vi "Memory.Pointer.Parameter Check.Size.0D.vi"(7 "source vi name":string, 8 "error in (no error)":errorcluster, 10 "required size":u64 format="%08x bytes", 11 "Pointer in":refnum<class "Memory.Pointer.lvclass">) -> (0 "error out":errorcluster, 2 "required size out":u64 format="%08x bytes", 3 "Pointer out":refnum<class "Memory.Pointer.lvclass">)   [LabVIEW 2016, in "Memory Manager.lvlib" / "Memory.Pointer.lvclass"]
uses:
  Memory.Pointer.lvclass
  Memory.Pointer.lvclass/Memory.Pointer.ctl
  Memory.Pointer.Errors.Out of Bounds.vi
  Submodules/Static Error Handling/Source/Library/VIs/Static Error Handling.Source Buffer.Write.String.vi
  Memory.Pointer.Errors.Write Pointer Size.vi
  Memory.Pointer.Errors.Create Error.vi
  Submodules/Static Error Handling/Source/Library/VIs/Static Error Handling.Source Buffer.Write.Numeric.Scalar.Base10.vi
  Submodules/Static Error Handling/Source/Library/VIs/Static Error Handling.Source Buffer.Write.Numeric.Scalar.Base10 (U64).vi
  Submodules/Static Error Handling/Source/Library/VIs/Static Error Handling.Error Cluster Constant.vi
  Submodules/Static Error Handling/Source/Library/VIs/Static Error Handling.Error Cluster Constant (256B).vi
  Submodules/Static Error Handling/Source/Library/VIs/Static Error Handling.Parameters.Status.Set.vi
  Submodules/Static Error Handling/Source/Library/VIs/Static Error Handling.Parameters.Code.Set.vi
  Submodules/Static Error Handling/Source/Library/VIs/Static Error Handling.Parameters.VI Source.Set.vi
  Constants/Memory.Constants.vi
  Constants/Memory.Constants.Library Name.vi
  Memory.Pointer.Errors.Get Info.vi
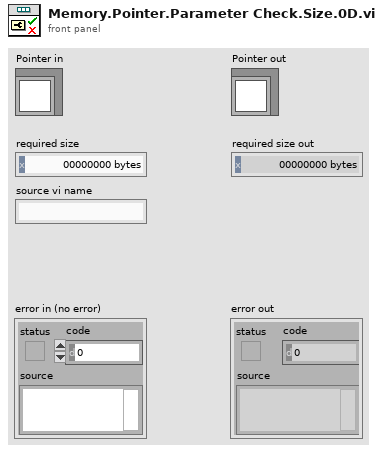
[diagram p1: front panel]
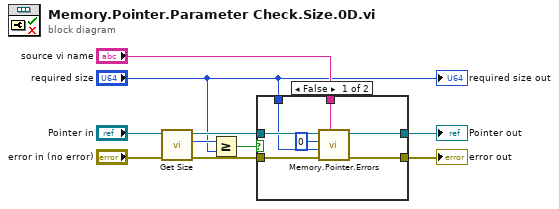
[diagram p0: block diagram]
diagram:
  n1 = call "Get Size.vi"("error in (no error)"="error in (no error)", "Pointer in"="Pointer in") -> ("error out"=w5:errorcluster, "size"=w8:u64, "Pointer out"=w3:refnum<class "Memory.Pointer.lvclass">)  [unwired: 7 in]
  n2 = Greater Or Equal?(x=w8, y="required size") -> (x >= y?=w4:bool)
  n3 = case shown="False" w4 {
    tunnel: w3 -> [w17 w18]
    tunnel: w5 -> [w15 w19]
    tunnel: [w14 w19] -> w10
    tunnel: [w16 w18] -> w9
    tunnel: "required size" -> [w13 _]
    tunnel: "source vi name" -> [w12 _]
    frame False {
      n4 = call-poly "Memory.Pointer.Errors.vi"("source vi name"=w12, "error in (no error)"=w15, "length"=w13, "offset"=u64 0, "pointer in"=w17) -> ("error out"=w14:errorcluster, "pointer out"=w16:refnum<class "Memory.Pointer.lvclass">)  [unwired: 5 in]
    }
    frame True {
    }
  }
  "error out" <- w10
  "Pointer out" <- w9
  "required size out" <- "required size"
